vi "Remove VI.vi"(8 "error in (no error)":errorcluster, 11 "WindowFrame in":refnum<class "WindowFrame.lvclass">) -> (0 "error out":errorcluster, 3 "WindowFrame out":refnum<class "WindowFrame.lvclass">)   [LabVIEW 2021, in "WindowFrame.lvlib" / "WindowFrame.lvclass"]
uses:
  WindowFrame.lvclass
  Action.ctl
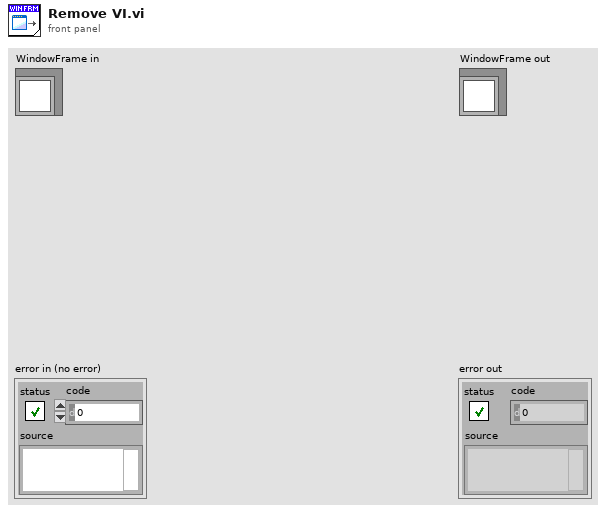
[diagram p1: front panel]
types:
  T1 = typedef "WindowFrame.lvlib/WindowFrame.lvclass/Action.ctl" = enum16{"Set Allow Runtime PopUp", "Set Behavior", "Set Closable", "Set Custom Title", "Set Highlight Return Button", "Set Is Frontmost", "Set Minimizable", "Set Minimum Size", "Set Monitor", "Set Resizable", "Set Panel Bounds", "Set Run VI Transparently", "Set Show Menu Bar", "Set State", "Set Title", "Set Title Bar Colors", "Set Title Bar Visible", "Set Transparancy", "Set Window Bounds", "Get Allow Runtime PopUp", "Get Behavior", "Get Closable", "Get Custom Title", "Get Highlight Return Button", "Get Is Frontmost", "Get Minimizable", "Get Minimum Size", "Get Monitor", "Get Panel Bounds", "Get Resizable", "Get Run VI Transparently", "Get Show Menu Bar", "Get State", "Get Title", "Get Title Bar Colors", "Get Title Bar Visible", "Get Transparancy", "Get Window Bounds", "--", "Center", "Close", "Open", "Run-Time Position:Centered", "Run-Time Position:Custom", "Run-Time Position:Get Position", "Run-Time Position:Maximized", "Run-Time Position:Minimized", "Run-Time Position:Unchanged", "---", "Insert VI", "Remove VI", "Insert VI Index", "Remove VI Index", "Exit"}
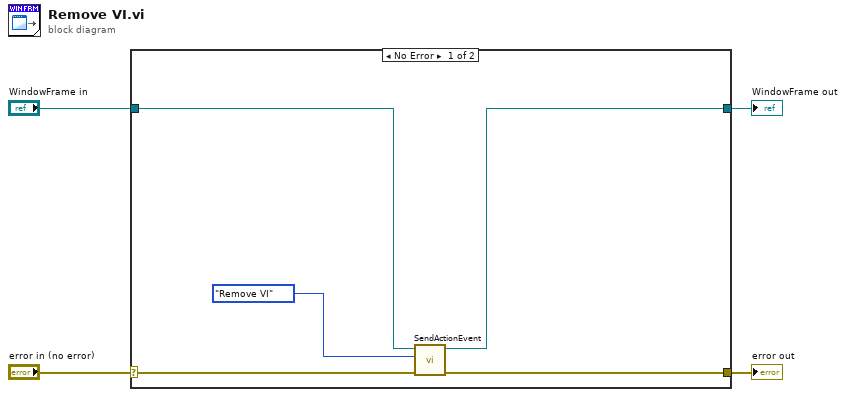
[diagram p0: block diagram]
diagram:
  n1 = case shown="No Error" "error in (no error)" {
    selector: "error in (no error)" -> [w9 w11]
    tunnel: [w8 w11] -> w3
    tunnel: [w7 w10] -> w1
    tunnel: "WindowFrame in" -> [w6 w10]
    frame No Error {
      n2 = call "SendActionEvent.vi"("error in (no error)"=w9, "Action"=Action."Remove VI", "WindowFrame in"=w6) -> ("error out"=w8:errorcluster, "WindowFrame out"=w7:refnum<class "WindowFrame.lvclass">)  [unwired: 7 in]
    }
    frame Error {
    }
  }
  "error out" <- w3
  "WindowFrame out" <- w1
